vi "simulate.vi"() -> ()   [LabVIEW 2017]
uses:
  040-typeDefs/Position.ctl
panel:
  out "XY Graph":cluster{"X":dbl, "Y":dbl}[](graph)
  in  "Numeric":i32=200
  in  "stop":bool
  in  "destination":T1
  in  "start":T1
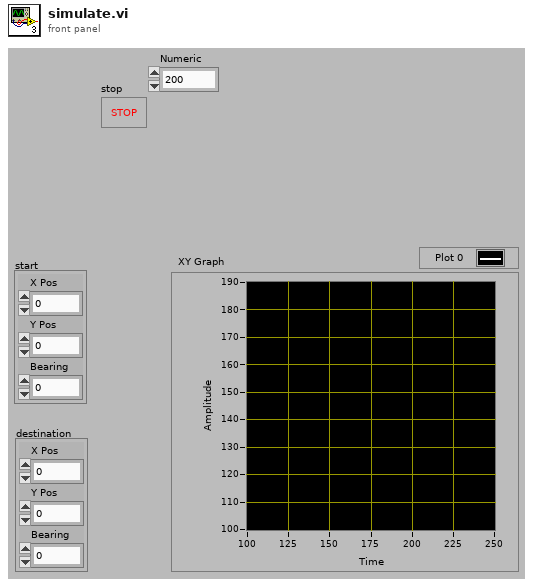
[diagram p1: front panel]
types:
  T1 = typedef "Position.ctl" = cluster{"X Pos":dbl, "Y Pos":dbl, "Bearing":dbl}
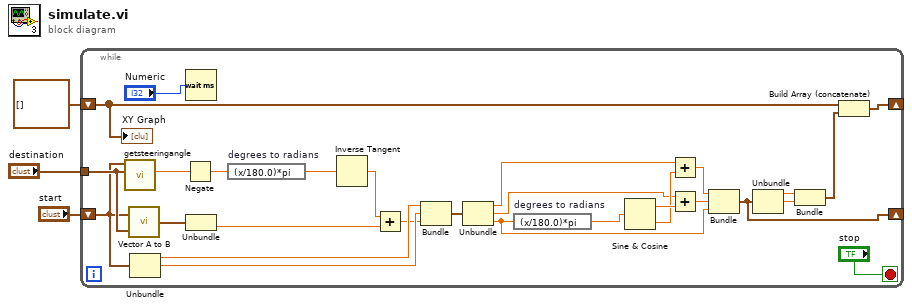
[diagram p0: block diagram]
diagram:
  n1 = while {
    tunnel: "destination" -> [w26]
    shift-right: [w7] -> _
    shift-left: "start" -> [w22]
    shift-right: [w9] -> _
    shift-left: cluster{dbl, dbl}[] [] -> [w4]
    stop <- "stop" stop-if-true
    n2 = call "getsteeringangle.vi"("Target Pose"=w26, "Current Robot"=w22) -> ("x-y"=w29:dbl)  [unwired: 9 in]
    n3 = call "Vector A to B.vi"("Destination"=w26, "Current"=w22) -> ("vector"=w25:cluster{dbl, "Bearing":dbl})
    n4 = Unbundle(w22) -> ("X Pos"=w21:dbl, "Y Pos"=w20:dbl)  [unwired: 1 out]
    n5 = Negate(x=w29) -> (-x=w28:dbl)
    n6 = Wait (ms)(milliseconds to wait="Numeric") -> ()  [unwired: 1 out]
    n7 = Unbundle(w25) -> ("Bearing"=w24:dbl)  [unwired: 1 out]
    n8 = expression code="(x/180.0)*pi" "degrees to radians"(w28) -> (w27:dbl)
    n9 = Inverse Tangent(1:w27) -> (0:w23:dbl)
    n10 = Add(x=w23, y=w24) -> (x+y=w19:dbl)
    n11 = Bundle("X Pos"=w21, "Y Pos"=w20, w19) -> (w18:cluster{"X Pos":dbl, "Y Pos":dbl, dbl})  [unwired: 1 in]
    n12 = Unbundle(w18) -> ("X Pos"=w13:dbl, "Y Pos"=w14:dbl, w10:dbl)
    n13 = expression code="(x/180.0)*pi" "degrees to radians"(w10) -> (w17:dbl)
    n14 = Sine & Cosine(0:w17) -> (1:w16:dbl, 2:w15:dbl)
    n15 = Add(x=w13, y=w15) -> (x+y=w12:dbl)
    n16 = Add(x=w14, y=w16) -> (x+y=w11:dbl)
    n17 = Bundle(w12, w11, w10) -> (w7:cluster{dbl, dbl, dbl})  [unwired: 1 in]
    n18 = Unbundle(w7) -> (w8:dbl, w6:dbl)  [unwired: 1 out]
    n19 = Bundle(w8, w6) -> (w5:cluster{dbl, dbl})  [unwired: 1 in]
    n20 = Build Array (concatenate)(w4, w5) -> (w9:cluster{dbl, dbl}[])
    "XY Graph" <- w4
  }
